vi "LegalJustify.vi"(8 "error in":errorcluster caption="错误输入", 10 "JustifyName":T1(ring), 11 "Setup":T2) -> (0 "error out":errorcluster caption="错误输出", 3 "OK？":bool)   [LabVIEW 2013]
uses:
  SetupCtl.ctl
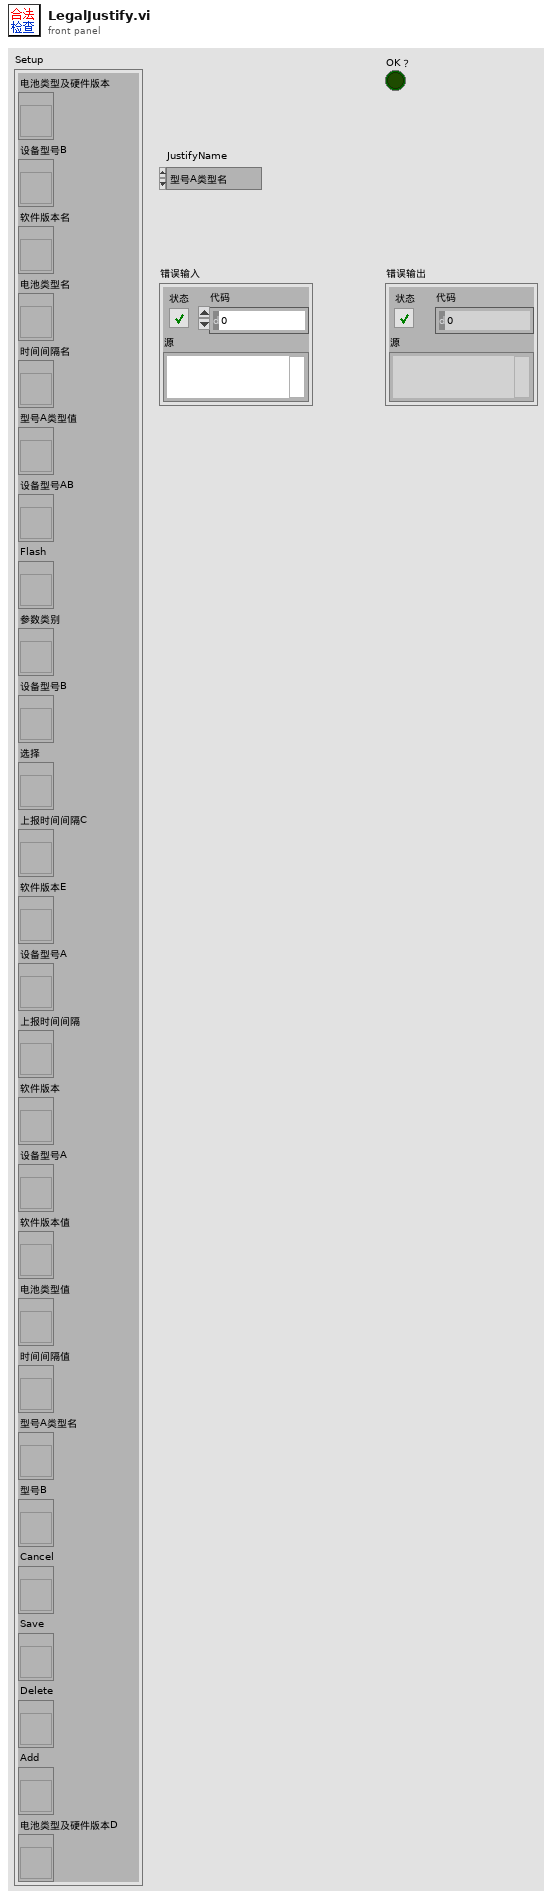
[diagram p1: front panel]
types:
  T1 = enum16{"型号A类型名", "型号A类型值", "型号B", "时间间隔名", "时间间隔值", "电池类型名", "电池类型值", "软件版本名", "软件版本值"}
  T2 = typedef "SetupCtl.ctl" = cluster{"电池类型及硬件版本":refnum<vi>, "设备型号B":refnum<vi>, "软件版本名":refnum<vi>, "电池类型名":refnum<vi>, "时间间隔名":refnum<vi>, "型号A类型值":refnum<vi>, "设备型号AB":refnum<vi>, "Flash":refnum<vi>, "参数类别":refnum<vi>, "设备型号B":refnum<vi>, "选择":refnum<vi>, "上报时间间隔C":refnum<vi>, "软件版本E":refnum<vi>, "设备型号A":refnum<vi>, "上报时间间隔":refnum<vi>, "软件版本":refnum<vi>, "设备型号A":refnum<vi>, "软件版本值":refnum<vi>, "电池类型值":refnum<vi>, "时间间隔值":refnum<vi>, "型号A类型名":refnum<vi>, "型号B":refnum<vi>, "Cancel":refnum<vi>, "Save":refnum<vi>, "Delete":refnum<vi>, "Add":refnum<vi>, "电池类型及硬件版本D":refnum<vi>}
  T3 = enum16{"型号AB", "型号A", "型号B", "上报时间间隔", "电池类型", "软件版本"}
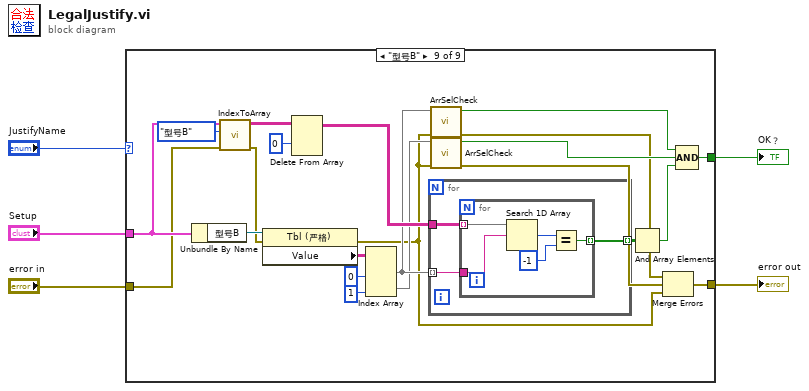
[diagram p0: block diagram]
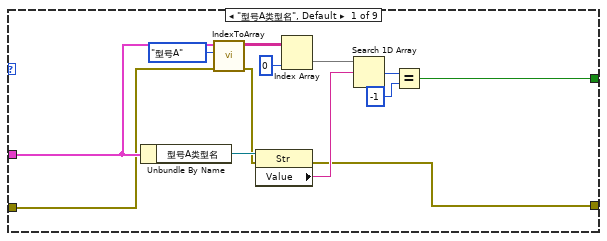
[diagram p2: hidden frame]
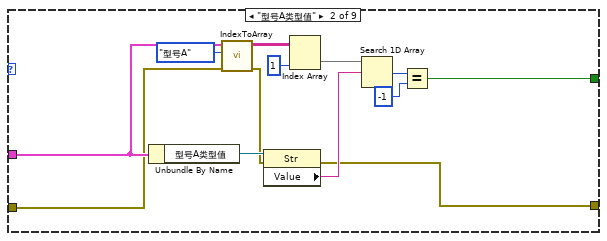
[diagram p3: hidden frame]
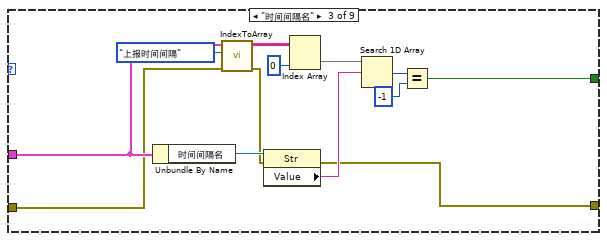
[diagram p4: hidden frame]
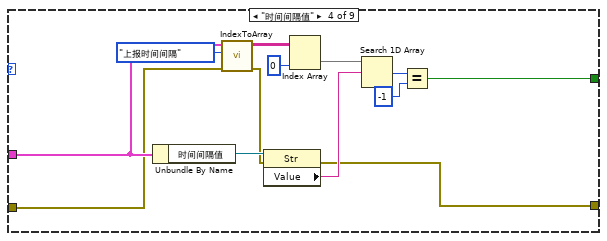
[diagram p5: hidden frame]
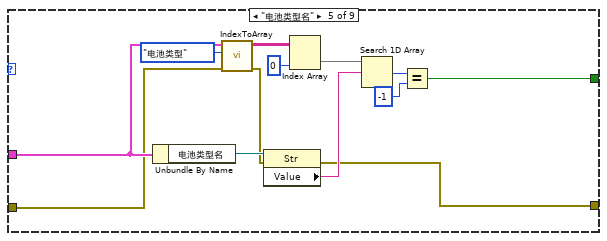
[diagram p6: hidden frame]
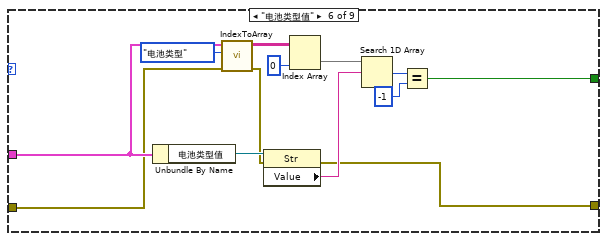
[diagram p7: hidden frame]
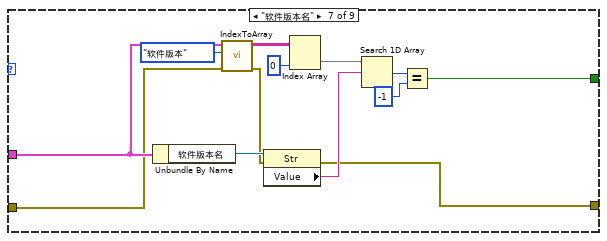
[diagram p8: hidden frame]
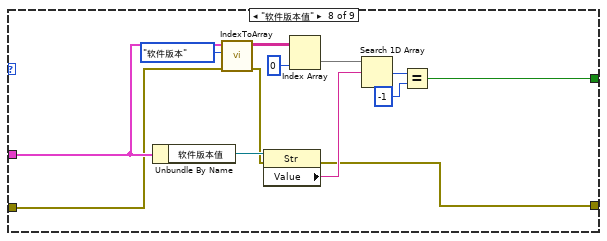
[diagram p9: hidden frame]
diagram:
  n1 = case shown="\"型号B\"" "JustifyName" {
    tunnel: "Setup" -> [w16 w29 w42 w55 w68 w81 w94 w107 w129]
    tunnel: [w9 w22 w35 w48 w61 w74 w87 w100 w114] -> w3
    tunnel: "error in" -> [w8 w21 w34 w47 w60 w73 w86 w99 w128]
    tunnel: [w6 w19 w32 w45 w58 w71 w84 w97 w113] -> w1
    frame "型号A类型名", Default {
      n2 = Unbundle By Name(w16) -> ("型号A类型名"=w18:refnum<vi>)
      n3 = call "IndexToArray.vi"("error in"=w8, "Extract"=T3."型号A", "Setup"=w16) -> ("error out"=w7:errorcluster, "Value"=w15:string[][])  [unwired: 7 in]
      n4 = property class="Str"(reference=w18, error in=w7) -> (error out=w6:errorcluster, "Value"=w12:string)  [unwired: 1 out]
      n5 = Index Array(array=w15, index (col)=0 ("禁用的索引 (列)")) -> (element=w13:string[])  [unwired: 1 in]
      n6 = Search 1D Array(1D array=w13, element=w12) -> (index of element=w11:i32)  [unwired: 1 in]
      n7 = Equal?(x=w11, y=-1) -> (x = y?=w9:bool)
    }
    frame "型号A类型值" {
      n8 = Unbundle By Name(w29) -> ("型号A类型值"=w31:refnum<vi>)
      n9 = call "IndexToArray.vi"("error in"=w21, "Extract"=T3."型号A", "Setup"=w29) -> ("error out"=w20:errorcluster, "Value"=w28:string[][])  [unwired: 7 in]
      n10 = property class="Str"(reference=w31, error in=w20) -> (error out=w19:errorcluster, "Value"=w25:string)  [unwired: 1 out]
      n11 = Index Array(array=w28, index (col)=1 ("禁用的索引 (列)")) -> (element=w26:string[])  [unwired: 1 in]
      n12 = Search 1D Array(1D array=w26, element=w25) -> (index of element=w24:i32)  [unwired: 1 in]
      n13 = Equal?(x=w24, y=-1) -> (x = y?=w22:bool)
    }
    frame "时间间隔名" {
      n14 = Unbundle By Name(w42) -> ("时间间隔名"=w44:refnum<vi>)
      n15 = call "IndexToArray.vi"("error in"=w34, "Extract"=T3."上报时间间隔", "Setup"=w42) -> ("error out"=w33:errorcluster, "Value"=w41:string[][])  [unwired: 7 in]
      n16 = property class="Str"(reference=w44, error in=w33) -> (error out=w32:errorcluster, "Value"=w38:string)  [unwired: 1 out]
      n17 = Index Array(array=w41, index (col)=0 ("禁用的索引 (列)")) -> (element=w39:string[])  [unwired: 1 in]
      n18 = Search 1D Array(1D array=w39, element=w38) -> (index of element=w37:i32)  [unwired: 1 in]
      n19 = Equal?(x=w37, y=-1) -> (x = y?=w35:bool)
    }
    frame "时间间隔值" {
      n20 = Unbundle By Name(w55) -> ("时间间隔值"=w57:refnum<vi>)
      n21 = call "IndexToArray.vi"("error in"=w47, "Extract"=T3."上报时间间隔", "Setup"=w55) -> ("error out"=w46:errorcluster, "Value"=w54:string[][])  [unwired: 7 in]
      n22 = property class="Str"(reference=w57, error in=w46) -> (error out=w45:errorcluster, "Value"=w51:string)  [unwired: 1 out]
      n23 = Index Array(array=w54, index (col)=0 ("禁用的索引 (列)")) -> (element=w52:string[])  [unwired: 1 in]
      n24 = Search 1D Array(1D array=w52, element=w51) -> (index of element=w50:i32)  [unwired: 1 in]
      n25 = Equal?(x=w50, y=-1) -> (x = y?=w48:bool)
    }
    frame "电池类型名" {
      n26 = Unbundle By Name(w68) -> ("电池类型名"=w70:refnum<vi>)
      n27 = call "IndexToArray.vi"("error in"=w60, "Extract"=T3."电池类型", "Setup"=w68) -> ("error out"=w59:errorcluster, "Value"=w67:string[][])  [unwired: 7 in]
      n28 = property class="Str"(reference=w70, error in=w59) -> (error out=w58:errorcluster, "Value"=w64:string)  [unwired: 1 out]
      n29 = Index Array(array=w67, index (col)=0 ("禁用的索引 (列)")) -> (element=w65:string[])  [unwired: 1 in]
      n30 = Search 1D Array(1D array=w65, element=w64) -> (index of element=w63:i32)  [unwired: 1 in]
      n31 = Equal?(x=w63, y=-1) -> (x = y?=w61:bool)
    }
    frame "电池类型值" {
      n32 = Unbundle By Name(w81) -> ("电池类型值"=w83:refnum<vi>)
      n33 = call "IndexToArray.vi"("error in"=w73, "Extract"=T3."电池类型", "Setup"=w81) -> ("error out"=w72:errorcluster, "Value"=w80:string[][])  [unwired: 7 in]
      n34 = property class="Str"(reference=w83, error in=w72) -> (error out=w71:errorcluster, "Value"=w77:string)  [unwired: 1 out]
      n35 = Index Array(array=w80, index (col)=0 ("禁用的索引 (列)")) -> (element=w78:string[])  [unwired: 1 in]
      n36 = Search 1D Array(1D array=w78, element=w77) -> (index of element=w76:i32)  [unwired: 1 in]
      n37 = Equal?(x=w76, y=-1) -> (x = y?=w74:bool)
    }
    frame "软件版本名" {
      n38 = Unbundle By Name(w94) -> ("软件版本名"=w96:refnum<vi>)
      n39 = call "IndexToArray.vi"("error in"=w86, "Extract"=T3."软件版本", "Setup"=w94) -> ("error out"=w85:errorcluster, "Value"=w93:string[][])  [unwired: 7 in]
      n40 = property class="Str"(reference=w96, error in=w85) -> (error out=w84:errorcluster, "Value"=w90:string)  [unwired: 1 out]
      n41 = Index Array(array=w93, index (col)=0 ("禁用的索引 (列)")) -> (element=w91:string[])  [unwired: 1 in]
      n42 = Search 1D Array(1D array=w91, element=w90) -> (index of element=w89:i32)  [unwired: 1 in]
      n43 = Equal?(x=w89, y=-1) -> (x = y?=w87:bool)
    }
    frame "软件版本值" {
      n44 = Unbundle By Name(w107) -> ("软件版本值"=w109:refnum<vi>)
      n45 = call "IndexToArray.vi"("error in"=w99, "Extract"=T3."软件版本", "Setup"=w107) -> ("error out"=w98:errorcluster, "Value"=w106:string[][])  [unwired: 7 in]
      n46 = property class="Str"(reference=w109, error in=w98) -> (error out=w97:errorcluster, "Value"=w103:string)  [unwired: 1 out]
      n47 = Index Array(array=w106, index (col)=0 ("禁用的索引 (列)")) -> (element=w104:string[])  [unwired: 1 in]
      n48 = Search 1D Array(1D array=w104, element=w103) -> (index of element=w102:i32)  [unwired: 1 in]
      n49 = Equal?(x=w102, y=-1) -> (x = y?=w100:bool)
    }
    frame "型号B" {
      n50 = Unbundle By Name(w129) -> ("型号B"=w131:refnum<vi>)
      n51 = call "IndexToArray.vi"("error in"=w128, "Extract"=T3."型号B", "Setup"=w129) -> ("error out"=w120:errorcluster, "Value"=w127:string[][])  [unwired: 7 in]
      n52 = property class="Tbl (严格)"(reference=w131, error in=w120) -> (error out=w110:errorcluster, "Value"=w125:string[][])  [unwired: 1 out]
      n53 = Delete From Array(array=w127, index (row)=0 ("索引 (行)")) -> (array with subset deleted=w122:string[][])  [unwired: 2 in, 1 out]
      n54 = Index Array(array=w125, index (col) #1=0 ("禁用的索引 (列)"), index (col) #2=1 ("索引 (列)")) -> (element #1=w119:string[], element #2=w118:string[])  [unwired: 2 in]
      n55 = for {
        tunnel: w119 -> [w133] mode=indexing
        tunnel: w122 -> [w134]
        tunnel: [w132] -> w123 mode=indexing
        n56 = for {
          tunnel: w134 -> [w135] mode=indexing
          tunnel: w133 -> [w139]
          tunnel: [w136] -> w132 mode=indexing
          n57 = Search 1D Array(1D array=w135, element=w139) -> (index of element=w138:i32)  [unwired: 1 in]
          n58 = Equal?(x=w138, y=-1) -> (x = y?=w136:bool)
        }
      }
      n59 = call "ArrSelCheck.vi"("error in"=w110, "ArrayIn"=w119) -> ("error out"=w112:errorcluster, "Repeat?"=w117:bool)  [unwired: 8 in]
      n60 = call "ArrSelCheck.vi"("error in"=w110, "ArrayIn"=w118) -> ("error out"=w111:errorcluster, "Repeat?"=w116:bool)  [unwired: 8 in]
      n61 = And Array Elements(Boolean array=w123) -> (logical AND=w115:bool)
      n62 = Merge Errors(w112, w111, w110) -> (w113:errorcluster)
      n63 = Compound Arithmetic op=AND(w117, w116, w115) -> (w114:bool)
    }
  }
  "OK？" <- w3
  "error out" <- w1
